vi "WeatherStationTCPTester.vi"() -> ()   [LabVIEW 2012]
panel:
  out "Converted":dbl[](array[numeric])=[20.166971916971917, 37.08943833943834, 837.1291208791208, 6.41025641025641, 100.0]
  out "Raw":dbl[](array[numeric])=[41794.0, 24301.0, 39103.0, 420.0, 482.0]
  out "Array":string[](array[string])=["$ 28673 M 00160 41794\r", "$ 28673 M 00260 24301\r", "$ 28673 M 00360 39103\r", "$ 28673 M 00270 00420\r", "$ 28673 M 00265 00482\r"]
  in  "Port":u16=4760
  in  "IPAddress":string="192.168.0.110"
  out "Error Out":errorcluster
  in  "Error In":errorcluster
  # "Temp\nRH\nPress\nMixing ratio\nAbsolute humidity"
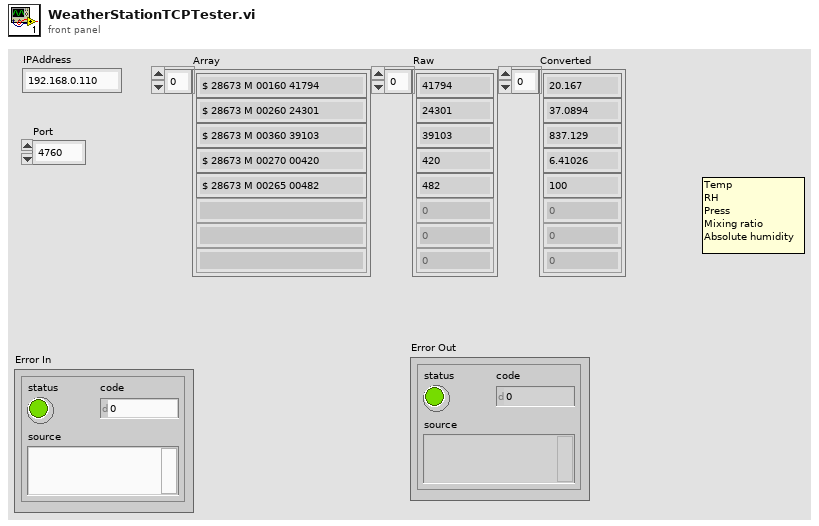
[diagram p1: front panel]
types:
  T1 = enum16{"Standard", "Buffered", "CRLF", "Immediate"}
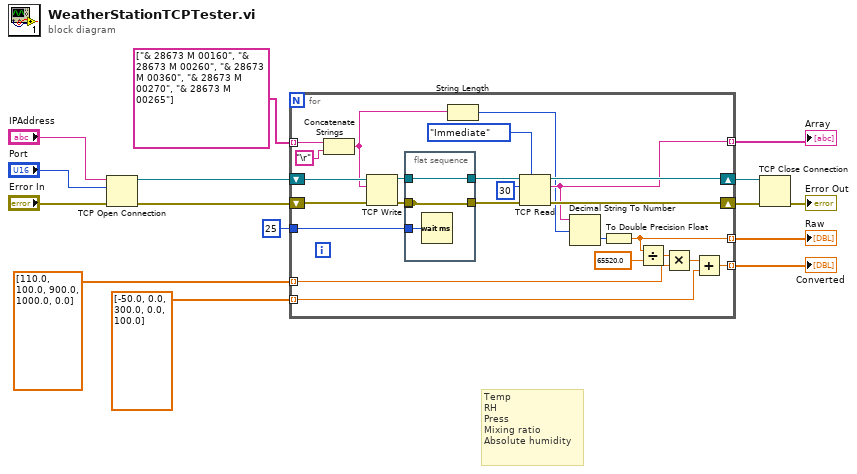
[diagram p0: block diagram]
diagram:
  # "Temp\nRH\nPress\nMixing ratio\nAbsolute humidity"
  n1 = TCP Open Connection(address="IPAddress", remote port or service name="Port", error in (no error)="Error In") -> (connection ID=w9:refnum<k5>, error out=w13:errorcluster)  [unwired: 2 in]
  n2 = for {
    tunnel: u32 25 ("wait (ms)") -> [w39]
    tunnel: string[] ["& 28673 M 00160", "& 28673 M 00260", "& 28673 M 00360", "& 28673 M 00270", "& 28673 M 00265"] -> [w37] mode=indexing
    shift-right: [w30] -> w8
    shift-left: w9 -> [w36]
    shift-right: [w31] -> w7
    shift-left: w13 -> [w35]
    tunnel: [w25] -> w5 mode=indexing
    tunnel: dbl[] [110.0, 100.0, 900.0, 1000.0, 0.0] -> [w17] mode=indexing
    tunnel: dbl[] [-50.0, 0.0, 300.0, 0.0, 100.0] -> [w16] mode=indexing
    tunnel: [w19] -> w2 mode=indexing
    tunnel: [w18] -> w1 mode=indexing
    n3 = Concatenate Strings(w37, "\r") -> (w26:string)
    n4 = TCP Write(connection ID=w36, data in=w26, error in (no error)=w35) -> (connection ID out=w34:refnum<k5>, error out=w33:errorcluster)  [unwired: 1 in, 1 out]
    n5 = flat-sequence {
      tunnel: [w41] -> w32
      tunnel: [w41] -> _
      tunnel: w39 -> [w42]
      tunnel: w34 -> [w40]
      tunnel: w33 -> [w41]
      tunnel: [w40] -> w29
      frame #0 {
        n6 = Wait (ms)(milliseconds to wait=w42) -> ()  [unwired: 1 out]
      }
    }
    n7 = String Length(string=w26) -> (length=w24:i32)
    n8 = TCP Read(connection ID=w29, bytes to read=u32 30 ("byte count"), error in (no error)=w32, 7:T1."Immediate" ("mode (standard)")) -> (connection ID out=w30:refnum<k5>, data out=w25:string, error out=w31:errorcluster)  [unwired: 1 in]
    n9 = Decimal String To Number(string=w25, offset=w24) -> (number=w23:i32)  [unwired: 1 in, 1 out]
    n10 = To Double Precision Float(number=w23) -> (double precision float=w19:dbl)
    n11 = Divide(x=w19, y=65520.0) -> (x/y=w21:dbl)
    n12 = Multiply(x=w21, y=w17) -> (x*y=w20:dbl)
    n13 = Add(x=w20, y=w16) -> (x+y=w18:dbl)
  }
  "Array" <- w5
  "Raw" <- w2
  "Converted" <- w1
  n14 = TCP Close Connection(connection ID=w8, error in (no error)=w7) -> (error out=→"Error Out":errorcluster)  [unwired: 1 in, 1 out]
